vi "时间计算.vi"(0 "跳变时间":u32) -> (1 "数值":dbl, 2 "连接的字符串":string)   [LabVIEW 2012]
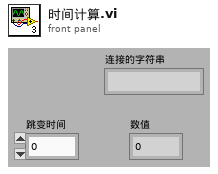
[diagram p1: front panel]
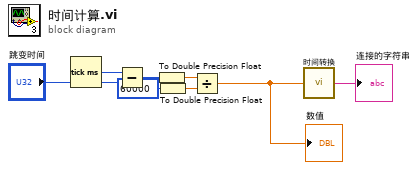
[diagram p0: block diagram]
diagram:
  n1 = Tick Count (ms)() -> (millisecond timer value=w6:u32)
  n2 = Subtract(x=w6, y="跳变时间") -> (x-y=w5:u32)
  n3 = To Double Precision Float(number=w5) -> (double precision float=w3:dbl)
  n4 = To Double Precision Float(number=u32 60000 ("y")) -> (double precision float=w2:dbl)
  n5 = Divide(x=w3, y=w2) -> (x/y=w8:dbl)
  "数值" <- w8
  n6 = call "时间转换.vi"("数值"=w8) -> ("字符串"=→"连接的字符串":string)
